vi "PostUUT_Action.vi"(8 "error in":errorcluster, 10 "TestResult":bool, 11 "GuiRef":T1) -> (0 "error out":errorcluster)   [LabVIEW 2013]
uses:
  Ctl/IOConfig.ctl
  GlobValue.vi
panel:
  out "IOConfig":T2={"DO"=[["钥匙keyin", "Dev2/port0/line0", "H", "DI"], ["遥控解锁", "Dev2/port0/line1", "H", "DI"], ["后背门", "Dev2/port0/line2", "H", "DI"], ["车门1", "Dev2/port0/line3", "H", "DI"]], "DI"=[["钥匙keyin", "Dev2/port0/line0", "H", "DI"], ["遥控解锁", "Dev2/port0/line1", "H", "DI"], ["后背门", "Dev2/port0/line2", "H", "DI"], ["车门1", "Dev2/port0/line3", "H", "DI"]]}
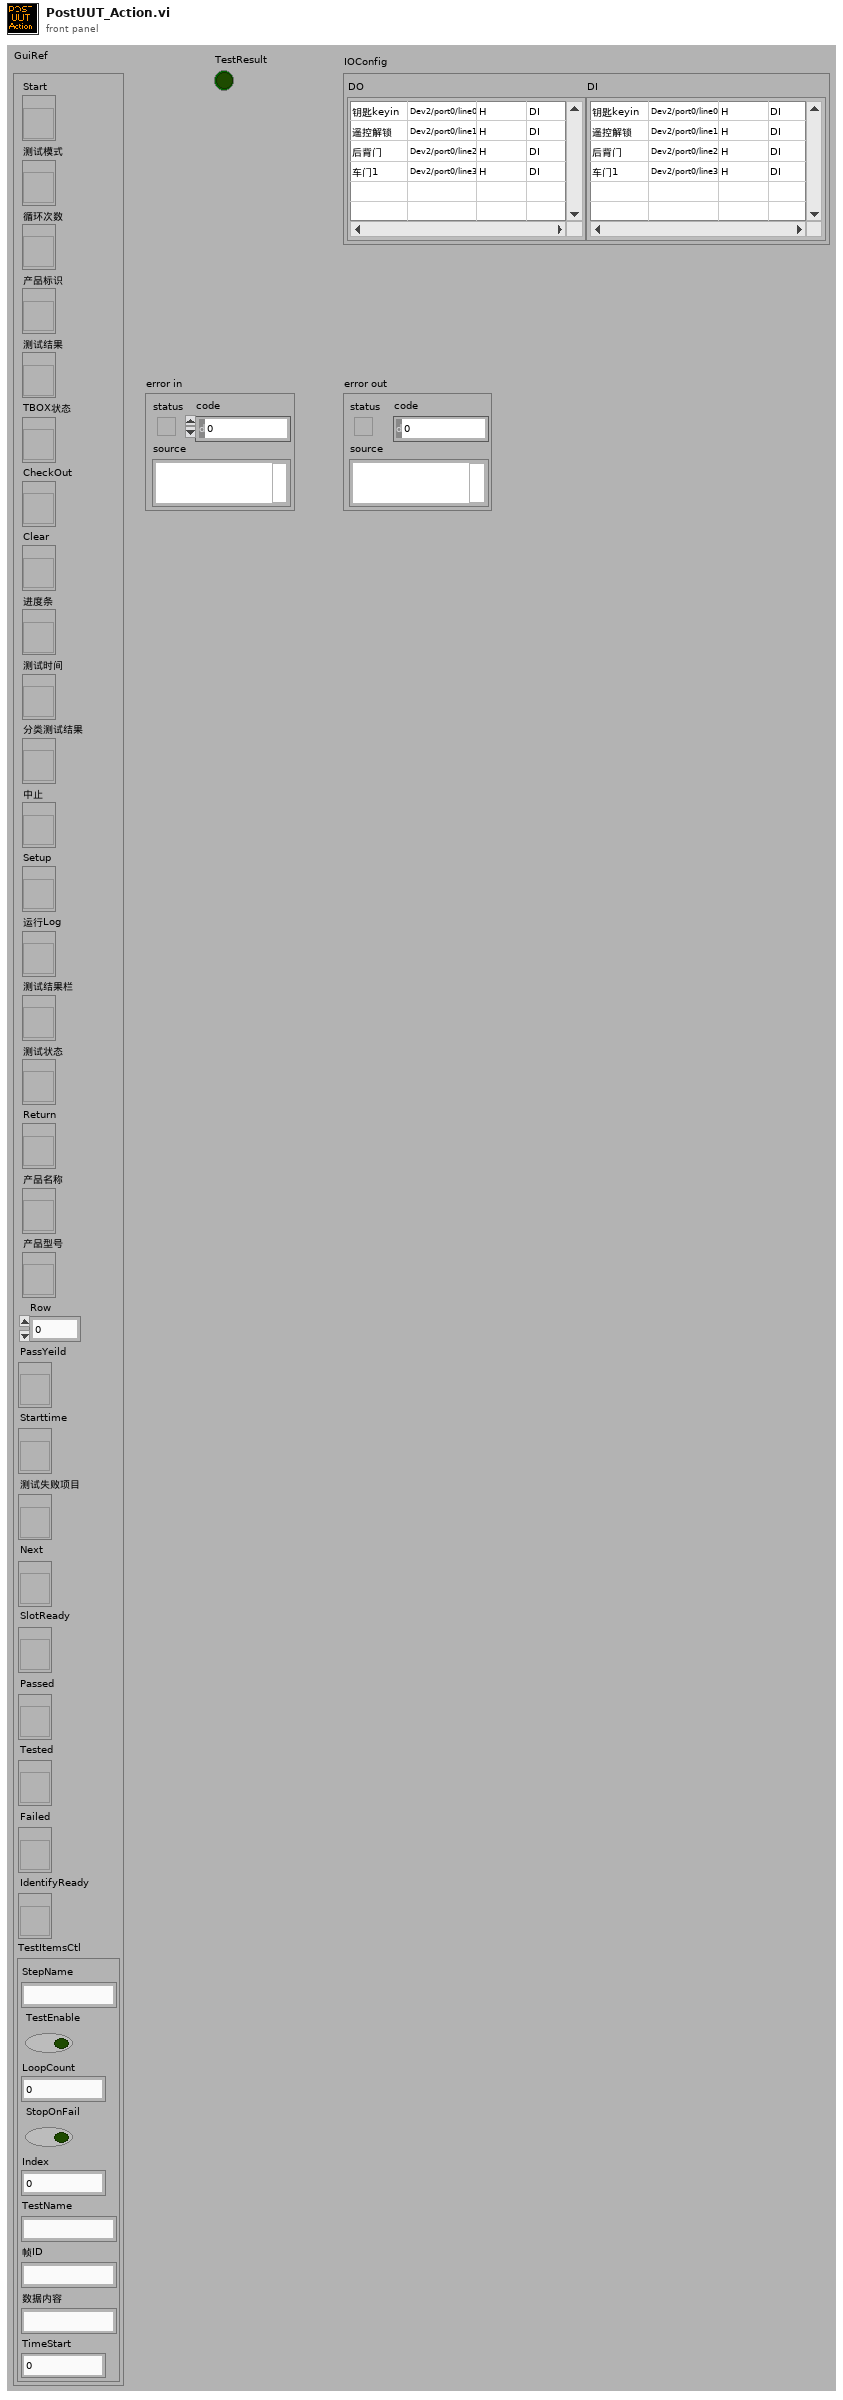
[diagram p1: front panel]
types:
  T1 = typedef "控件.ctl" = cluster{"Start":refnum<vi>, "测试模式":refnum<vi>, "循环次数":refnum<vi>, "产品标识":refnum<vi>, "测试结果":refnum<vi>, "TBOX状态":refnum<vi>, "CheckOut":refnum<vi>, "Clear":refnum<vi>, "进度条":refnum<vi>, "测试时间":refnum<vi>, "分类测试结果":refnum<vi>, "中止":refnum<vi>, "Setup":refnum<vi>, "运行Log":refnum<vi>, "测试结果栏":refnum<vi>, "测试状态":refnum<vi>, "Return":refnum<vi>, "产品名称":refnum<vi>, "产品型号":refnum<vi>, "Row":i32, "PassYeild":refnum<vi>, "Starttime":refnum<vi>, "测试失败项目":refnum<vi>, "Next":refnum<vi>, "SlotReady":refnum<vi>, "Passed":refnum<vi>, "Tested":refnum<vi>, "Failed":refnum<vi>, "IdentifyReady":refnum<vi>, "TestItemsCtl":cluster{"StepName":string, "TestEnable":bool, "LoopCount":u32, "StopOnFail":bool, "Index":u32, "TestName":string, "帧ID":string, "数据内容":string, "TimeStart":u32}}
  T2 = typedef "IOConfig.ctl" = cluster{"DO":string[][], "DI":string[][]}
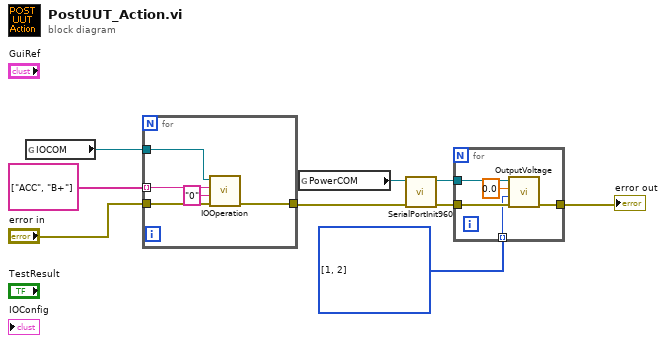
[diagram p0: block diagram]
diagram:
  w1 = i32[] [1, 2] items=["Channel 1"=1, "Channel 2"=2]
  n1 = global read "GlobValue.vi" "IOCOM"() -> (w8:refnum<visa-resource-name>)
  n2 = for "For循环" {
    tunnel: string[] ["ACC", "B+"] -> [w14] mode=indexing
    tunnel: w8 -> [w13]
    tunnel: "error in" -> [w11]
    tunnel: [w10] -> w3
    n3 = call "IOOperation.vi"("error in"=w11, "Value"="0", "Channel"=w14, "Com"=w13) -> ("error out"=w10:errorcluster)  [unwired: 5 in, 2 out]
  }
  n4 = global read "GlobValue.vi" "PowerCOM"() -> (w6:refnum<visa-resource-name>)
  n5 = call "SerialPortInit960.vi"("错误输入"=w3, "COMIn"=w6) -> ("错误输出"=w4:errorcluster, "COMOut"=w5:refnum<visa-resource-name>)  [unwired: 8 in]
  n6 = for {
    tunnel: w5 -> [w19]
    tunnel: w4 -> [w18]
    tunnel: [w17] -> w2
    tunnel: w1 -> [w15] mode=indexing
    n7 = call "OutputVoltage.vi"("error in"=w18, "Channel"=w15, "Voltage Level"=0.0, "VISAin"=w19) -> ("error out"=w17:errorcluster)  [unwired: 5 in, 2 out]
  }
  "error out" <- w2
